vi "Link Test Channels.vi"(7 "gRPC ID in":T4, 8 "error in (no error)":errorcluster, 10 "Channels":T1[](array[typedef]), 11 "CIFCorePlugin in":refnum<class "CIFCorePlugin.lvclass">) -> (0 "error out":errorcluster, 3 "CIFCorePlugin out":refnum<class "CIFCorePlugin.lvclass">)   [LabVIEW 2021, in "Template_Test_Helpers.lvlib"]
uses:
  Template_Test_Helpers.lvlib
  <vilib>/gRPC/LabVIEW gRPC Library/Shared/grpcId.ctl
  <vilib>/CIF Foundation/CIF Core/CIFCore/Grpc/CIFCoreChannel_client/RPC Messages/cif_channelcore_Channel.ctl
  <vilib>/CIF Foundation/CIF Core/CIFCore/Grpc/CIFCoreChannel_client/RPC Messages/cif_channelcore_Direction.ctl
  <vilib>/CIF Foundation/CIF Core/CIFCore/Grpc/CIFCoreChannel_client/RPC Messages/cif_channelcore_PATTERN.ctl
  <vilib>/CIF Foundation/CIF Core/CIFCore/Class/CIFCorePlugin.lvclass
  <vilib>/CIF Foundation/CIF Core/CIFCore/Class/CIFCorePlugin.lvclass/CIFCorePlugin.ctl
  <vilib>/CIF Foundation/CIF Channels Core/ChannelCommon/typedef/New FIFO Instance Configuration.ctl
  <vilib>/CIF Foundation/CIF Channels Core/CIFChannels/CIFChannels.lvclass/CIFChannels.ctl
  <vilib>/CIF Foundation/CIF Core/CIFCore/Common/Typedef/FIFO Publisher.ctl
  <vilib>/CIF Foundation/CIF Core/CIFCore/Grpc/CIFCoreChannel_client/RPC Messages/cif_channelcore_ConnectSubscriber.ctl
  <vilib>/CIF Foundation/CIF Channels Core/CIFChannels/Accessors/Read Direction.vi
  <vilib>/CIF Foundation/CIF Channels Core/CIFChannels/Accessors/Read Name.vi
  <vilib>/CIF Foundation/CIF Channels Core/CIFChannels/Accessors/Read Custom Config Data.vi
  <vilib>/CIF Foundation/CIF Core/CIFCore/Class/Accessors/Read Channel Array.vi
  <vilib>/CIF Foundation/CIF Core/CIFCore/Class/Accessors/Write Channel Array.vi
  <vilib>/CIF Foundation/CIF Utilities/DataTypes/Flatten Unflatten/Unflatten U64.vi
  <vilib>/CIF Foundation/CIF Channels Core/CIFChannels/CIFChannels.lvclass
  <vilib>/CIF Foundation/CIF Core/CIFCore/Grpc/CIFCoreWrapper/CIFCoreWrapper.lvlib
  <vilib>/CIF Foundation/CIF Channels Core/ChannelCommon/ChannelCommon.lvlib
  <vilib>/CIF Foundation/CIF Core/CIFCore/Grpc/CIFCoreChannel_client/CIFCoreChannel_client.lvlib
  <vilib>/CIF Foundation/CIF Core/CIFCore/Common/CIFCoreCommon.lvlib
  <vilib>/gRPC/LabVIEW gRPC Library/grpc-lvsupport-release.lvlib
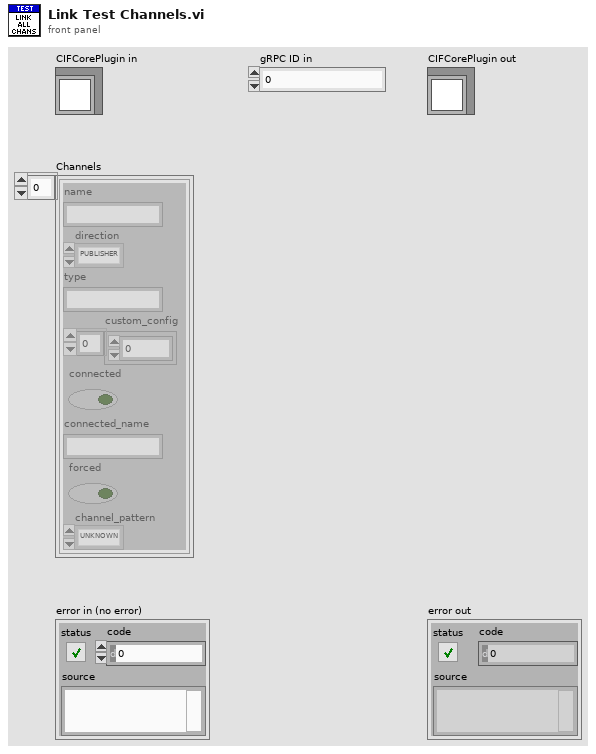
[diagram p1: front panel]
types:
  T1 = typedef "CIFCoreChannel_client.lvlib/cif_channelcore_Channel.ctl" = cluster{"name":string, "direction":T2, "type":string, "custom_config":u8[], "connected":bool, "connected_name":string, "forced":bool, "channel_pattern":T3}
  T2 = typedef "CIFCoreChannel_client.lvlib/cif_channelcore_Direction.ctl" = enum32{"PUBLISHER", "SUBSCRIBER"}
  T3 = typedef "CIFCoreChannel_client.lvlib/cif_channelcore_PATTERN.ctl" = enum32{"UNKNOWN", "TAG", "FIFO", "MULTIFIFO", "BACKPRESSUREFIFO"}
  T4 = typedef "grpc-lvsupport-release.lvlib/grpcId.ctl" = u64
  T5 = typedef "ChannelCommon.lvlib/New FIFO Instance Configuration.ctl" = cluster{"Backpressure":bool, "Bytes/Message Override":u32, "Messages/FIFO Override":u32, "Custom Data":u8[]}
  T6 = typedef "CIFCoreCommon.lvlib/FIFO Publisher.ctl" = cluster{"Publisher Name":string, "New FIFO Instance Config":T5}
  T7 = typedef "CIFCoreChannel_client.lvlib/cif_channelcore_ConnectSubscriber.ctl" = cluster{"subscriber_name":string, "publisher_name":string, "custom_connect":u8[]}
  T8 = typedef "CIFChannels.lvclass/Direction.ctl" = enum16{"Publisher", "Subscriber"}
  T9 = typedef "ChannelCommon.lvlib/FIFO Config.ctl" = cluster{"Max Bytes/Msg":u64, "Max Msg/FIFO":u64, "Flags":u64, "Custom Data":u8[]}
  T10 = typedef "ChannelCommon.lvlib/FIFO Flags.ctl" = cluster{"Backpressure":bool}
  T11 = typedef "ChannelCommon.lvlib/New FIFO Instance Response.ctl" = cluster{"Publisher":string, "Custom Data":u8[]}
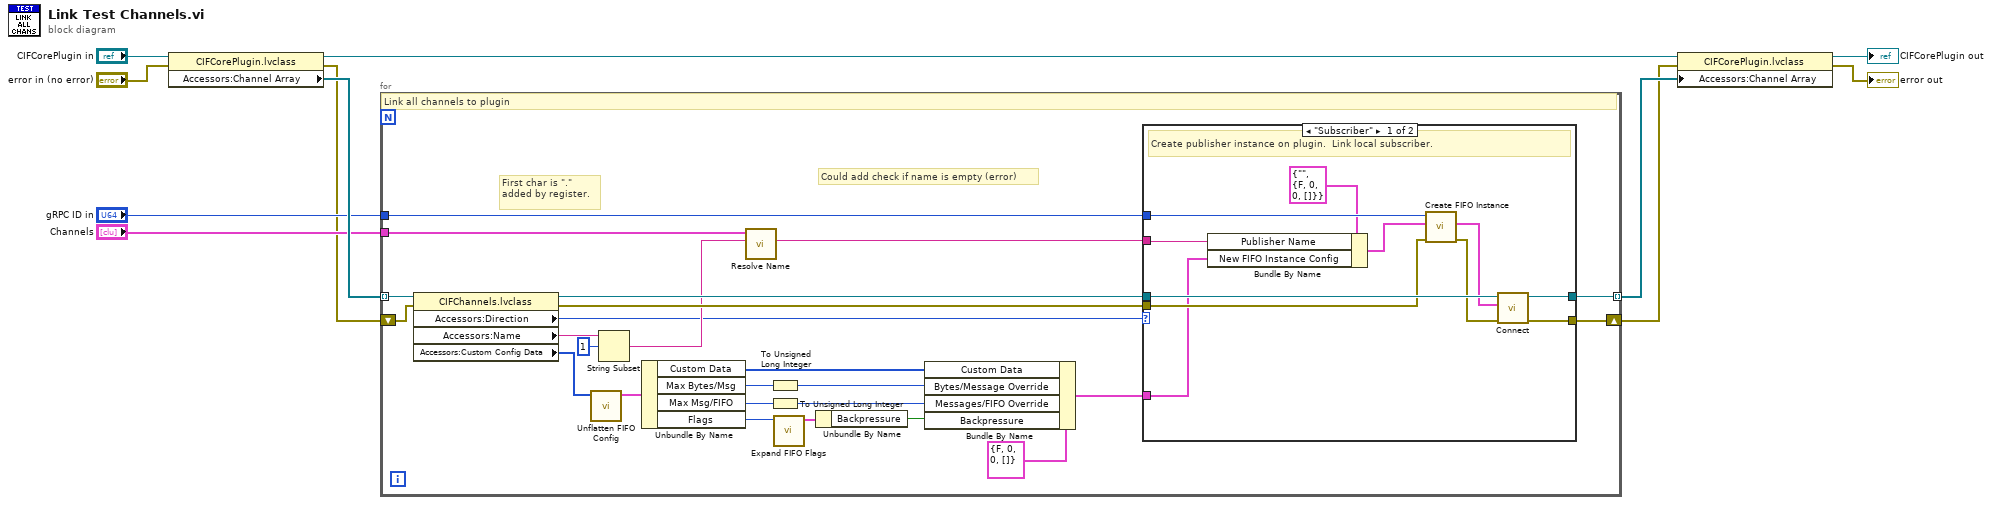
[diagram p0: block diagram]
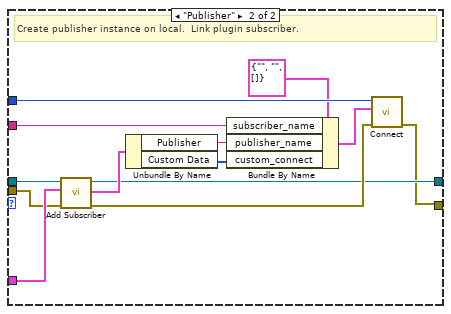
[diagram p2: hidden frame]
diagram:
  n1 = property class="CIFCorePlugin.lvclass"(reference="CIFCorePlugin in", error in="error in (no error)") -> (reference out=w5:refnum<class "CIFCorePlugin.lvclass">, error out=w6:errorcluster, "Accessors:Channel Array"=w10:refnum<class "CIFChannels.lvclass">[])
  n2 = for {
    tunnel: w10 -> [w36] mode=indexing
    tunnel: "Channels" -> [w33]
    tunnel: "gRPC ID in" -> [w32]
    tunnel: [w29] -> w4 mode=indexing
    shift-right: [w28] -> w2
    shift-left: w6 -> [w31]
    # "Could add check if name is empty (error)"
    # "First char is \".\" added by register."
    # "Link all channels to plugin"
    n3 = property class="CIFChannels.lvclass"(reference=w36, error in=w31) -> (reference out=w35:refnum<class "CIFChannels.lvclass">, error out=w30:errorcluster, "Accessors:Direction"=w16:T8, "Accessors:Name"=w14:string, "Accessors:Custom Config Data"=w34:u8[])
    n4 = call <vilib>:"Unflatten FIFO Config.vi"("Flattened Data in"=w34) -> ("FIFO Config out"=w27:T9)  [unwired: 9 in, 1 out]
    n5 = String Subset(string=w14, offset (0)=1) -> (substring=w17:string)  [unwired: 1 in]
    n6 = Unbundle By Name(w27) -> ("Custom Data"=w21:u8[], "Max Bytes/Msg"=w25:u64, "Max Msg/FIFO"=w24:u64, "Flags"=w26:u64)
    n7 = call <vilib>:"Resolve Name.vi"("Name in"=w17, "Channels"=w33) -> ("Name out"=w13:string)  [unwired: 7 in, 2 out]
    n8 = To Unsigned Long Integer(number=w25) -> (unsigned 32bit integer=w20:u32)
    n9 = To Unsigned Long Integer(number=w24) -> (unsigned 32bit integer=w19:u32)
    n10 = call <vilib>:"Expand FIFO Flags.vi"("FIFO Flags"=w26) -> ("Flags"=w23:T10)  [unwired: 10 in]
    n11 = Unbundle By Name(w23) -> ("Backpressure"=w22:bool)
    n12 = Bundle By Name(cluster=T5 {"Backpressure"=FALSE, "Bytes/Message Override"=0, "Messages/FIFO Override"=0, "Custom Data"=[]} ("New FIFO Instance Config"), "Custom Data"=w21, "Bytes/Message Override"=w20, "Messages/FIFO Override"=w19, "Backpressure"=w22) -> (w12:T5)
    n13 = case shown="\"Subscriber\"" w16 {
      tunnel: w35 -> [w47 w60]
      tunnel: w32 -> [w46 w59]
      tunnel: w30 -> [w45 w52]
      tunnel: [w44 w50] -> w29
      tunnel: [w43 w49] -> w28
      tunnel: w12 -> [w38 w58]
      tunnel: w13 -> [w39 w48]
      frame "Subscriber" {
        # "Create publisher instance on plugin.  Link local subscriber."
        n14 = Bundle By Name(cluster=T6 {"Publisher Name"="", "New FIFO Instance Config"={"Backpressure"=FALSE, "Bytes/Message Override"=0, "Messages/FIFO Override"=0, "Custom Data"=[]}} ("New Publisher"), "Publisher Name"=w39, "New FIFO Instance Config"=w38) -> (w37:T6)
        n15 = call <vilib>:"Create FIFO Instance.vi"("error in"=w45, "New Publisher"=w37, "gRPC ID"=w46) -> ("error out"=w42:errorcluster, "FIFO Instance"=w41:T11)  [unwired: 6 in, 1 out]
        n16 = call-dynamic <vilib>:"Connect.vi"("error in (no error)"=w42, "Connection"=w41, "CIFChannels in"=w47) -> ("error out"=w43:errorcluster, "CIFChannels out"=w44:refnum<class "CIFChannels.lvclass">)  [unwired: 7 in]
      }
      frame "Publisher" {
        # "Create publisher instance on local.  Link plugin subscriber."
        n17 = call-dynamic "Add Subscriber.vi"("error in (no error)"=w52, "New FIFO Instance Config"=w58, "CIFChannels in"=w60) -> ("error out"=w51:errorcluster, "New FIFO Instance"=w56:T11, "CIFChannels out"=w50:refnum<class "CIFChannels.lvclass">)  [unwired: 6 in]
        n18 = Unbundle By Name(w56) -> ("Publisher"=w55:string, "Custom Data"=w54:u8[])
        n19 = Bundle By Name(cluster=T7 {"subscriber_name"="", "publisher_name"="", "custom_connect"=[]} ("Connection"), "subscriber_name"=w48, "publisher_name"=w55, "custom_connect"=w54) -> (w53:T7)
        n20 = call <vilib>:"Connect.vi"("error in"=w51, "Connection"=w53, "gRPC ID"=w59) -> ("error out"=w49:errorcluster)  [unwired: 7 in, 1 out]
      }
    }
  }
  n21 = property class="CIFCorePlugin.lvclass"(reference=w5, error in=w2, "Accessors:Channel Array"=w4) -> (reference out=→"CIFCorePlugin out":refnum<class "CIFCorePlugin.lvclass">, error out=→"error out":errorcluster)
